vi "Configure Trigger Holdoff.vi"(8 "error in (no error)":errorcluster, 9 "Trigger Holdoff (60E-9)":dbl=6e-08 format="%^#_6g", 10 "Trigger Type (0: Edge)":u16(ring) items=["Edge", "Glitch", "Pattern", "CAN", "Duration", "IIC", "LIN", "Sequence", "SPI", "TV", "USB"], 11 "VISA resource name":refnum<visa-resource-name>) -> (0 "error out":errorcluster, 3 "VISA resource name out":refnum<visa-resource-name>)   [LabVIEW 2017, in "Agilent 6000 Series.lvlib"]
doc: "This VI configures the holdoff time of the trigger. After the scope detects a trigger, the trigger holdoff time is the amount of time before the scope begins looking for another trigger event. \n\n<B>NOTE:</B>\n It is not necessary to call this VI to change the trigger type, but the type will indeed change after this VI is called. To ensure correct use of this VI, make sure that the Trigger Type chosen in this VI corresponds with the type of the VI called from the Configure Trigger Poly VI."
uses:
  <instrlib>/Agilent 6000 Series/Agilent 6000 Series.lvlib
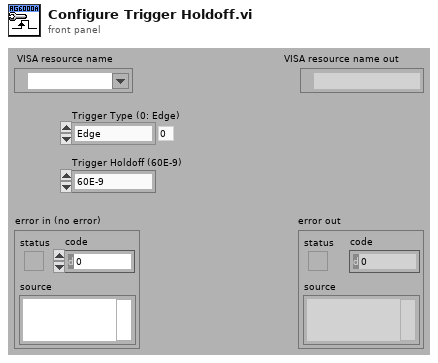
[diagram p1: front panel]
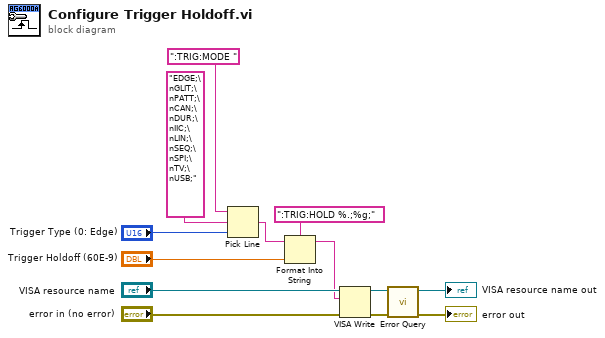
[diagram p0: block diagram]
diagram:
  n1 = Pick Line(string ("")=":TRIG:MODE ", multi-line string="EDGE;\nGLIT;\nPATT;\nCAN;\nDUR;\nIIC;\nLIN;\nSEQ;\nSPI;\nTV;\nUSB;", line index="Trigger Type (0: Edge)") -> (output string=w1:string)
  n2 = Format Into String(format string=":TRIG:HOLD %.;%g;" ("Level Command"), initial string=w1, "Trigger Holdoff (60E-9)") -> (resulting string=w5:string)  [unwired: 1 in, 1 out]
  n3 = VISA Write(VISA resource name="VISA resource name", write buffer=w5, error in (no error)="error in (no error)") -> (VISA resource name out=w9:refnum<visa-resource-name>, error out=w8:errorcluster)  [unwired: 1 out]
  n4 = call <instrlib>:"Error Query.vi"("error in (no error)"=w8, "VISA resource name"=w9) -> ("error out"=→"error out":errorcluster, "VISA resource name out"=→"VISA resource name out":refnum<visa-resource-name>)  [unwired: 6 in, 2 out]
